vi "Thev-Find Null.vi"(0 "Path":path, 7 "Freq":dbl) -> (4 "Path dup":path, 8 "Null freq (Hz)":dbl)   [LabVIEW 2015]
uses:
  Utility VIs/Math VIs/dB to Linear (1D).vi
  <vilib>/Analysis/NI_AALPro.lvlib
  <vilib>/Analysis/NI_AAL_SigProc.lvlib
panel:
  out "XY Graph 2":cluster{"Frequency (Hz)":dbl[], "Mag":dbl[]}(graph)
  out "XY Graph":cluster{"Frequency (Hz)":dbl[], "Mag":dbl[]}(graph)
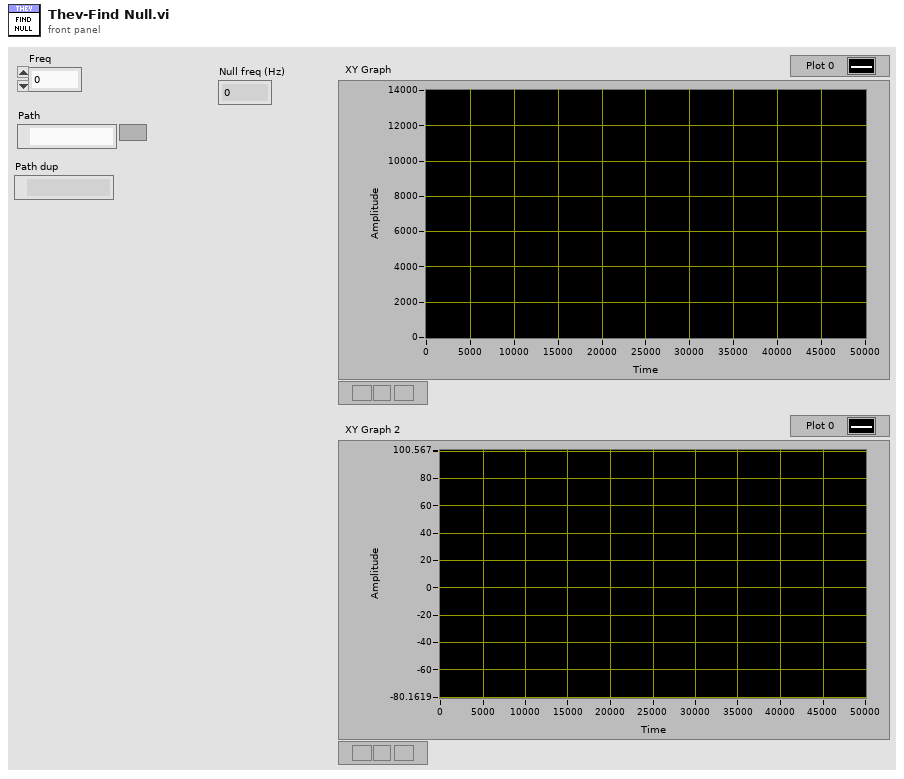
[diagram p1: front panel]
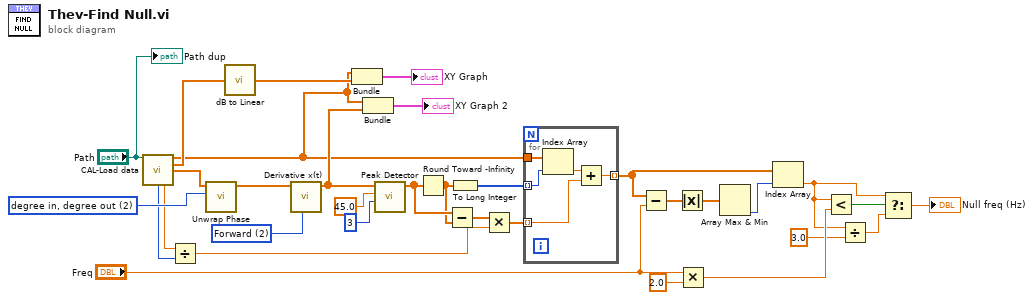
[diagram p0: block diagram]
diagram:
  w24 = u16 2 items=["2nd Order Central", "4th Order Central", "Forward", "Backward"] ("method")
  w28 = 2 items=["radian in, radian out", "radian in, degree out", "degree in, degree out", "degree in, radian out"] ("phase unit")
  n1 = call "CAL-Load data.vi"("user path"="Path") -> ("Frequency (Hz)"=w21:dbl[], "Mag"=w32:dbl[], "Phase"=w29:dbl[], "npts"=w14:i32, "Fs (Hz)"=w15:dbl)  [unwired: 7 in, 3 out]
  n2 = Divide(x=w15, y=w14) -> (x/y=w9:dbl)
  n3 = call <vilib>:"Unwrap Phase.vi"("phase unit"=w28, "Phase"=w29) -> ("Unwrapped Phase"=w22:dbl[])  [unwired: 8 in, 1 out]
  n4 = call-poly "dB to Linear.vi"("dB"=w32) -> ("linear"=w27:dbl[])
  n5 = call <vilib>:"Derivative x(t).vi"("method"=w24, "X"=w22) -> ("dX/dt"=w23:dbl[])  [unwired: 8 in, 1 out]
  n6 = Bundle("Frequency (Hz)"=w21, "linear"=w27) -> (→"XY Graph":cluster{"Frequency (Hz)":dbl[], "linear":dbl[]})  [unwired: 1 in]
  n7 = Bundle("Frequency (Hz)"=w21, "dX/dt"=w23) -> (→"XY Graph 2":cluster{"Frequency (Hz)":dbl[], "dX/dt":dbl[]})  [unwired: 1 in]
  n8 = call <vilib>:"Peak Detector.vi"("width"=3, "threshold"=45.0, "X"=w23) -> ("Locations"=w13:dbl[])  [unwired: 4 in, 4 out]
  n9 = Round Toward -Infinity(1:w13) -> (0:w12:dbl[])
  n10 = Subtract(x=w13, y=w12) -> (x-y=w11:dbl[])
  n11 = To Long Integer(number=w12) -> (32bit integer=w20:i32[])
  n12 = Multiply(x=w11, y=w9) -> (x*y=w10:dbl[])
  n13 = for {
    tunnel: w21 -> [w38]
    tunnel: w20 -> [w37] mode=indexing
    tunnel: [w35] -> w17 mode=indexing
    tunnel: w10 -> [w34] mode=indexing
    n14 = Index Array(array=w38, index=w37) -> (element=w36:dbl)
    n15 = Add(x=w36, y=w34) -> (x+y=w35:dbl)
  }
  n16 = Subtract(x=w17, y="Freq") -> (x-y=w19:dbl[])
  n17 = Absolute Value(x=w19) -> (abs(x)=w18:dbl[])
  n18 = Multiply(x="Freq", y=2.0) -> (x*y=w6:dbl)
  n19 = Array Max & Min(array=w18) -> (min index (indices)=w16:i32)  [unwired: 3 out]
  n20 = Index Array(array=w17, index=w16) -> (element=w4:dbl)
  n21 = Less?(x=w4, y=w6) -> (x < y?=w5:bool)
  n22 = Divide(x=w4, y=3.0) -> (x/y=w2:dbl)
  n23 = Select(t=w4, s=w5, f=w2) -> (s? t:f=→"Null freq (Hz)":dbl)
  "Path dup" <- "Path"
